vi "updateRfUnits.vi"(8 "error in (no error)":errorcluster, 11 "StaticOutputEditor in":refnum<class "StaticOutputEditor.lvclass">) -> (0 "error out":errorcluster, 3 "StaticOutputEditor out":refnum<class "StaticOutputEditor.lvclass">)   [LabVIEW 2011, in "Views.lvlib" / "ScriptEditor.lvlib" / "StaticOutputEditor.lvclass"]
uses:
  StaticOutputEditor.lvclass
  StaticOutputEditor.lvclass/StaticOutputEditor.ctl
  Tools/DatabaseHelpers/Database Objects/ChannelArray/ChannelArray.lvclass
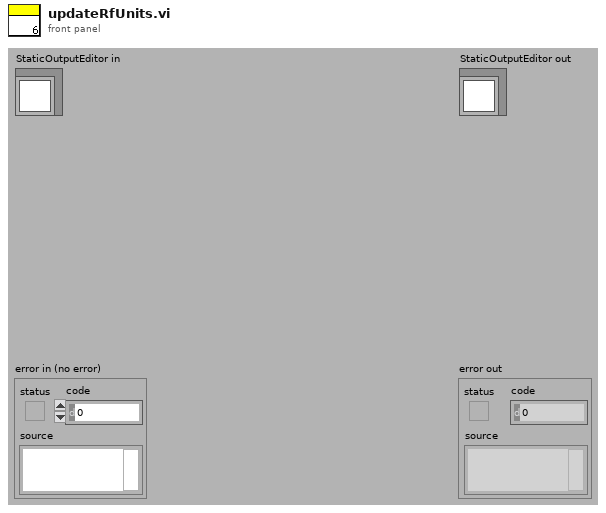
[diagram p1: front panel]
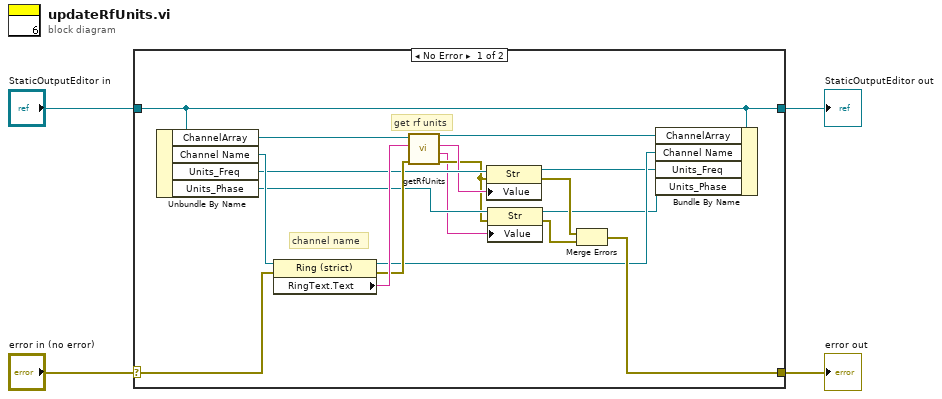
[diagram p0: block diagram]
diagram:
  n1 = case shown="No Error" "error in (no error)" {
    selector: "error in (no error)" -> [w21 w24]
    tunnel: [w10 w24] -> w3
    tunnel: [w9 w23] -> w1
    tunnel: "StaticOutputEditor in" -> [w9 w23]
    frame No Error {
      # "get rf units"
      # "channel name"
      n2 = Unbundle By Name(w9) -> ("ChannelArray"=w20:refnum<class "ChannelArray.lvclass">, "Channel Name"=w22:refnum<vi>, "Units_Freq"=w17:refnum<vi>, "Units_Phase"=w15:refnum<vi>)
      n3 = property class="Ring (strict)"(reference=w22, error in=w21) -> (reference out=w7:refnum<vi>, error out=w18:errorcluster, "RingText.Text"=w19:string)
      n4 = call "getRfUnits.vi"("error in (no error)"=w18, "channel_name"=w19, "ChannelArray in"=w20) -> ("error out"=w14:errorcluster, "phase_units"=w13:string, "freq_units"=w16:string, "ChannelArray out"=w8:refnum<class "ChannelArray.lvclass">)  [unwired: 5 in]
      n5 = property class="Str"(reference=w17, error in=w14, "Value"=w16) -> (reference out=w6:refnum<vi>, error out=w12:errorcluster)
      n6 = property class="Str"(reference=w15, error in=w14, "Value"=w13) -> (reference out=w5:refnum<vi>, error out=w11:errorcluster)
      n7 = Merge Errors(w12, w11) -> (w10:errorcluster)
      n8 = Bundle By Name(cluster=w9, "ChannelArray"=w8, "Channel Name"=w7, "Units_Freq"=w6, "Units_Phase"=w5) -> ()  [unwired: 1 out]
    }
    frame Error {
    }
  }
  "error out" <- w3
  "StaticOutputEditor out" <- w1
